vi "After Launch Init.vi"(8 "error in (no error)":errorcluster, 11 "CS++DeviceActor in":refnum<class "CS++DeviceActor.lvclass">) -> (0 "error out":errorcluster, 3 "CS++DeviceActor out":refnum<class "CS++DeviceActor.lvclass">)   [LabVIEW 2013, in "CS++DeviceActor.lvlib" / "CS++DeviceActor.lvclass"]
doc: "Use <b>Pre Launch init.vi</b> method for sanity checks that are supposed to prevent the actor from launching if they fail. Use <B>this</B> method instead to initialize this actor when it has been activated. A corresponding high priority message will become dispatched before the <B>Actor Core.vi</b> is called.\n\n<b>Derived classed should call the parent methode first</b> and their own initialization code after.\n\nRefer also to the ongoing discussion at https://decibel.ni.com/content/message/57394#57394."
uses:
  CS++DeviceActor.lvclass
  Classes/CS++ProcessVariables/SVConnection/SVConnection.lvclass
  CS++BaseActor/CS++BaseActor.lvclass
  CS++DeviceActor.lvclass/CS++DeviceActor.ctl
  Classes/CS++ProcessVariables/PVConnection/PVConnection.lvclass/PVConnection.ctl
  <vilib>/ActorFramework/Actor/Actor.lvclass/Actor.ctl
  <vilib>/ActorFramework/Message Enqueuer/Message Enqueuer.lvclass/Message Enqueuer.ctl
  CS++BaseActor/CS++BaseActor.lvclass/CS++BaseActor.ctl
  CS++DeviceActor Messages/Initialize Device Msg/Initialize Device Msg.lvclass/Initialize Device Msg.ctl
  CS++BaseActor Messages/Launch GUI Msg/Launch GUI Msg.lvclass/Launch GUI Msg.ctl
  <vilib>/ActorFramework/Message Enqueuer/Init from Existing Queue.vi
  <vilib>/ActorFramework/Message Enqueuer/Enqueue.vi
  <vilib>/ActorFramework/Message Priority Queue/Priority Enqueue.vi
  <vilib>/ActorFramework/Message Enqueuer/Message Enqueuer.lvclass
  CS++DeviceActor Messages/Initialize Device Msg/Initialize Device Msg.lvclass
  CS++DeviceActor Messages/Selftest Device Msg/Selftest Device Msg.lvclass
  CS++BaseActor Messages/Launch GUI Msg/Launch GUI Msg.lvclass
  Classes/CS++ProcessVariables/PVConnection/PVConnection.lvclass
  <vilib>/ActorFramework/Actor/Actor.lvclass
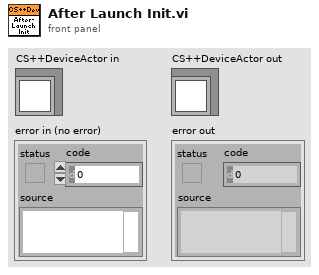
[diagram p1: front panel]
types:
  T1 = cluster{"Write Access":enum8{"Allowed", "Required", "None"}, "Read Access":enum8{"Allowed", "Required", "None"}}
  T2 = cluster{"Resource Name":string, "Driver Revision":string, "Firmware Revision":string, "Self-Test Result Code":string, "Self-Test Result Message":string, "Error Code":string, "Error Message":string}
  T3 = cluster{"[0]":refnum<class "SVConnection.lvclass">, "[1]":refnum<class "SVConnection.lvclass">, "[2]":refnum<class "SVConnection.lvclass">, "[3]":refnum<class "SVConnection.lvclass">, "[4]":refnum<class "SVConnection.lvclass">, "[5]":refnum<class "SVConnection.lvclass">, "[6]":refnum<class "SVConnection.lvclass">}
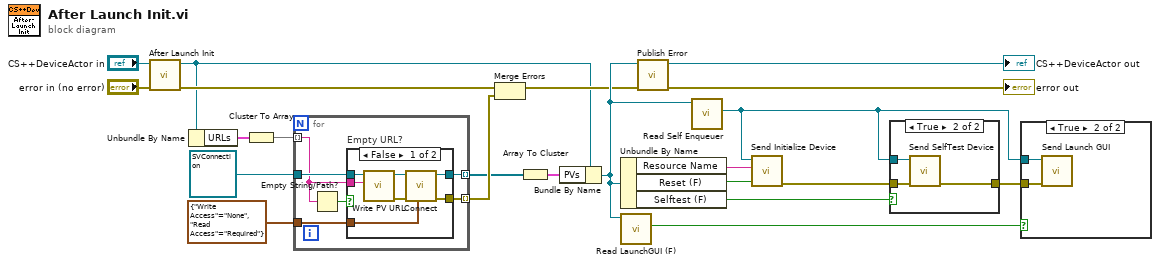
[diagram p0: block diagram]
diagram:
  n1 = call-parent "After Launch Init.vi"("error in (no error)"="error in (no error)", "CS++BaseActor in"="CS++DeviceActor in") -> ("error out"=w4:errorcluster, "CS++BaseActor out"=w2:refnum<class "CS++DeviceActor.lvclass">)  [unwired: 8 in]
  n2 = Unbundle By Name(w2) -> ("URLs"=w5:T2)
  n3 = Cluster To Array(cluster=w5) -> (array=w7:string[])
  n4 = for {
    tunnel: w7 -> [w24] mode=indexing
    tunnel: refnum<class "SVConnection.lvclass"> refnum ("CS++ProcessVariables.lvlib:SVConnection.lvclass") -> [w28]
    tunnel: T1 {"Write Access"=enum."None", "Read Access"=enum."Required"} ("Access") -> [w27]
    tunnel: [w26] -> w10 mode=indexing
    tunnel: [w23] -> w18 mode=indexing
    n5 = Empty String/Path?(string/path=w24) -> (empty?=w25:bool)
    n6 = case "Empty URL?" shown="False" w25 {
      tunnel: w28 -> [w35 w36]
      tunnel: w24 -> [w34 _]
      tunnel: w27 -> [w31 _]
      tunnel: [w30 w36] -> w26
      tunnel: [w29 _] -> w23
      frame False {
        n7 = call "Write PV URL.vi"("PV URL"=w34, "PVConnection in"=w35) -> ("error out"=w32:errorcluster, "PVConnection out"=w33:refnum<class "SVConnection.lvclass">)  [unwired: 8 in]
        n8 = call-dynamic "Connect.vi"("Access"=w31, "error in (no error)"=w32, "PVConnection in"=w33) -> ("error out"=w29:errorcluster, "PVConnection out"=w30:refnum<class "SVConnection.lvclass">)  [unwired: 7 in]
      }
      frame True {
      }
    }
  }
  n9 = Merge Errors(w4, w18) -> (w17:errorcluster)
  n10 = Array To Cluster(array=w10) -> (cluster=w6:T3)
  n11 = Bundle By Name(cluster=w2, "PVs"=w6) -> (w19:refnum<class "CS++DeviceActor.lvclass">)
  n12 = Unbundle By Name(w19) -> ("Resource Name"=w11:string, "Reset (F)"=w12:bool, "Selftest (F)"=w14:bool)
  n13 = call "Read LaunchGUI (F).vi"("CS++BaseActor in"=w19) -> ("LaunchGUI (F)"=w20:bool)  [unwired: 8 in, 2 out]
  n14 = call "Publish Error.vi"("error in (no error)"=w17, "CS++DeviceActor in"=w19) -> ("error out"=→"error out":errorcluster, "CS++DeviceActor out"=→"CS++DeviceActor out":refnum<class "CS++DeviceActor.lvclass">)  [unwired: 8 in]
  n15 = call <vilib>:"Read Self Enqueuer.vi"("Actor"=w19) -> ("Self Enqueuer"=w15:refnum<class "Message Enqueuer.lvclass">)  [unwired: 10 in]
  n16 = call "Send Initialize Device.vi"("Reset (F)"=w12, "Resource Name"=w11, "Message Enqueuer"=w15) -> ("error out"=w13:errorcluster)  [unwired: 7 in, 1 out]
  n17 = case shown="True" w14 {
    tunnel: w15 -> [_ w40]
    tunnel: w13 -> [w37 w39]
    tunnel: [w37 w38] -> w16
    frame False {
    }
    frame True {
      n18 = call "Send SelfTest Device.vi"("error in (no error)"=w39, "Message Enqueuer"=w40) -> ("error out"=w38:errorcluster)  [unwired: 8 in, 1 out]
    }
  }
  n19 = case shown="True" w20 {
    tunnel: w15 -> [_ w42]
    tunnel: w16 -> [_ w41]
    frame False {
    }
    frame True {
      n20 = call "Send Launch GUI.vi"("error in (no error)"=w41, "Message Enqueuer"=w42) -> ()  [unwired: 8 in, 2 out]
    }
  }
